vi "Start Trigger.vi"   [LabVIEW 2017, in "Sefram DAS220.lvlib"]
doc: "Start recording on condition."
uses:
  <instrlib>/Sefram DAS220/Sefram DAS220.lvlib
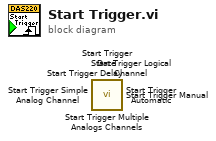
[diagram p0: block diagram]
diagram:
  n1 = call <instrlib>:"Start Trigger Multiple Analogs Channels.vi"() -> ()  [unwired: 10 in, 2 out]
  n2 = call <instrlib>:"Start Trigger Logical Channel.vi"() -> ()  [unwired: 10 in, 2 out]
  n3 = call <instrlib>:"Start Trigger Simple Analog Channel.vi"() -> ()  [unwired: 10 in, 2 out]
  n4 = call <instrlib>:"Start Trigger Manual.vi"() -> ()  [unwired: 10 in, 2 out]
  n5 = call <instrlib>:"Start Trigger Delay.vi"() -> ()  [unwired: 10 in, 2 out]
  n6 = call <instrlib>:"Start Trigger Date.vi"() -> ()  [unwired: 10 in, 2 out]
  n7 = call <instrlib>:"Start Trigger Automatic.vi"() -> ()  [unwired: 10 in, 2 out]
